vi "Device Activate.vi"(6 "Activate Mode":T1, 8 "error in (no error)":errorcluster, 10 "IED":string, 11 "SCADA in":refnum<class "SCADA.lvclass">) -> (0 "error out":errorcluster, 3 "SCADA out":refnum<class "SCADA.lvclass">)   [LabVIEW 2015, in "SCADA Core.lvlib" / "SCADA.lvclass"]
uses:
  SCADA.lvclass
  IED Actor/IED/Controls/Device Activate Mode Select.ctl
  Controls/Queue Selector.ctl
  IED Actor/IED Messages/Device Activate Msg/Device Activate Msg.lvclass/Device Activate Msg.ctl
  <vilib>/ActorFramework/Message Enqueuer/Message Enqueuer.lvclass/Message Enqueuer.ctl
  SCADA Abstract Messages/Device Action Status Msg/Device Action Status.ctl
  <vilib>/ActorFramework/Actor/Actor.lvclass/Actor.ctl
  SCADA Response Messages/Return Device Activate Status Msg/Return Device Activate Status Msg.lvclass/Return Device Activate Status Msg.ctl
  <vilib>/ActorFramework/Message Enqueuer/Enqueue.vi
  <vilib>/ActorFramework/Message Enqueuer/Init from Existing Queue.vi
  <vilib>/ActorFramework/Message Priority Queue/Priority Enqueue.vi
  IED Actor/IED Messages/Device Activate Msg/Device Activate Msg.lvclass
  <vilib>/ActorFramework/Message Enqueuer/Message Enqueuer.lvclass
  SCADA Response Messages/Return Device Activate Status Msg/Return Device Activate Status Msg.lvclass
  <vilib>/ActorFramework/Actor/Actor.lvclass
  SCADA Abstract Messages/Device Action Status Msg/Device Action Status Msg.lvclass
  IED Actor/IED/IED.lvclass
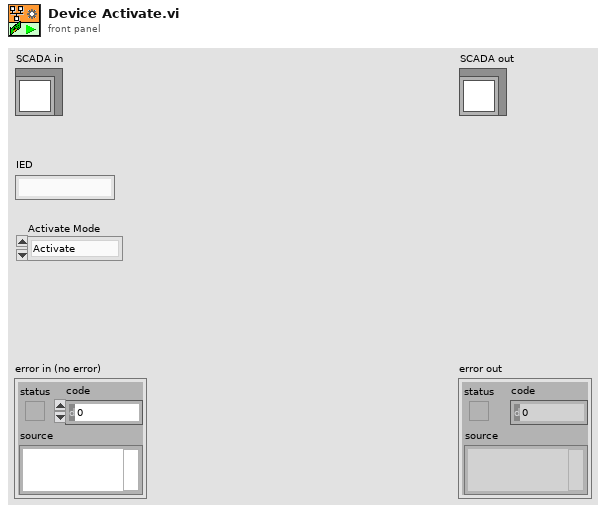
[diagram p1: front panel]
types:
  T1 = typedef "IED Actor.lvlib/IED.lvclass/Device Activate Mode Select.ctl" = enum16{"Activate", "Blackstart", "Individual"}
  T2 = typedef "SCADA Core.lvlib/SCADA.lvclass/Queue Selector.ctl" = enum16{"IEDs", "PV", "Generators", "Wind", "Storage", "Relays"}
  T3 = typedef "SCADA Core.lvlib/Device Action Status Msg.lvclass/Device Action Status.ctl" = enum16{"Success", "Failure"}
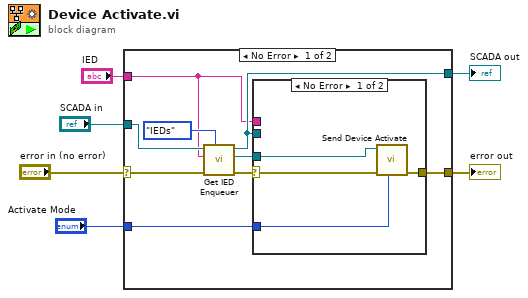
[diagram p0: block diagram]
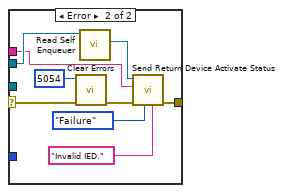
[diagram p2: hidden frame]
diagram:
  n1 = case shown="No Error" "error in (no error)" {
    selector: "error in (no error)" -> [w13 w30]
    tunnel: [w8 w30] -> w5
    tunnel: [w10 w29] -> w3
    tunnel: "SCADA in" -> [w15 w29]
    tunnel: "IED" -> [w9 _]
    tunnel: "Activate Mode" -> [w7 _]
    frame No Error {
      n2 = call "Get IED Enqueuer.vi"("Queue (IEDs)"=Queue_Selector."IEDs" ("Queue"), "error in (no error)"=w13, "IED Name"=w9, "SCADA in"=w15) -> ("error out"=w12:errorcluster, "IED Enqueuer"=w11:refnum<class "Message Enqueuer.lvclass">, "SCADA out"=w10:refnum<class "SCADA.lvclass">)  [unwired: 5 in]
      n3 = case shown="No Error" w12 {
        selector: w12 -> [w18 w26]
        tunnel: w11 -> [w19 _]
        tunnel: [w17 w22] -> w8
        tunnel: w10 -> [_ w28]
        tunnel: w9 -> [_ w25]
        tunnel: w7 -> [w16 _]
        frame No Error {
          n4 = call "Send Device Activate.vi"("Activate Mode"=w16, "error in (no error)"=w18, "Message Enqueuer"=w19) -> ("error out"=w17:errorcluster)  [unwired: 7 in, 1 out]
        }
        frame Error {
          n5 = call <vilib>:"Clear Errors.vi"("error in (no error)"=w26, "specific error code to clear (0: all)"=5054) -> ("error out"=w21:errorcluster)  [unwired: 4 in, 1 out]
          n6 = call <vilib>:"Read Self Enqueuer.vi"("Actor"=w28) -> ("Self Enqueuer"=w27:refnum<class "Message Enqueuer.lvclass">)  [unwired: 10 in]
          n7 = call "Send Return Device Activate Status.vi"("error string"="Invalid IED.", "Status"=Device_Action_Status."Failure", "error in (no error)"=w21, "IED Name"=w25, "Message Enqueuer"=w27) -> ("error out"=w22:errorcluster)  [unwired: 5 in, 1 out]
        }
      }
    }
    frame Error {
    }
  }
  "error out" <- w5
  "SCADA out" <- w3
